vi "6b8pointdft.vi"() -> ()   [LabVIEW 2013]
uses:
  <vilib>/Analysis/2dsp.llb/Real FFT.vi
  <vilib>/Analysis/NI_AALPro.lvlib
panel:
  out "XY Graph":cluster{i32[], dbl[]}(graph)
  out "Waveform Graph 1+2":dynamicdata(graph)
  out "Waveform Graph 2":dynamicdata(graph)
  out "Waveform Graph 1":dynamicdata(graph)
  in  "Amplitude 2":dbl=1.0 caption="Amplitude"
  in  "Frequency 2":dbl=10.1 caption="Frequency"
  in  "Frequency":dbl=10.1
  in  "Amplitude":dbl=1.0
  # "G SURESH\n23A91A0417\nECE-A"
  # "6B) FAST FOURIER TRANSFROM"
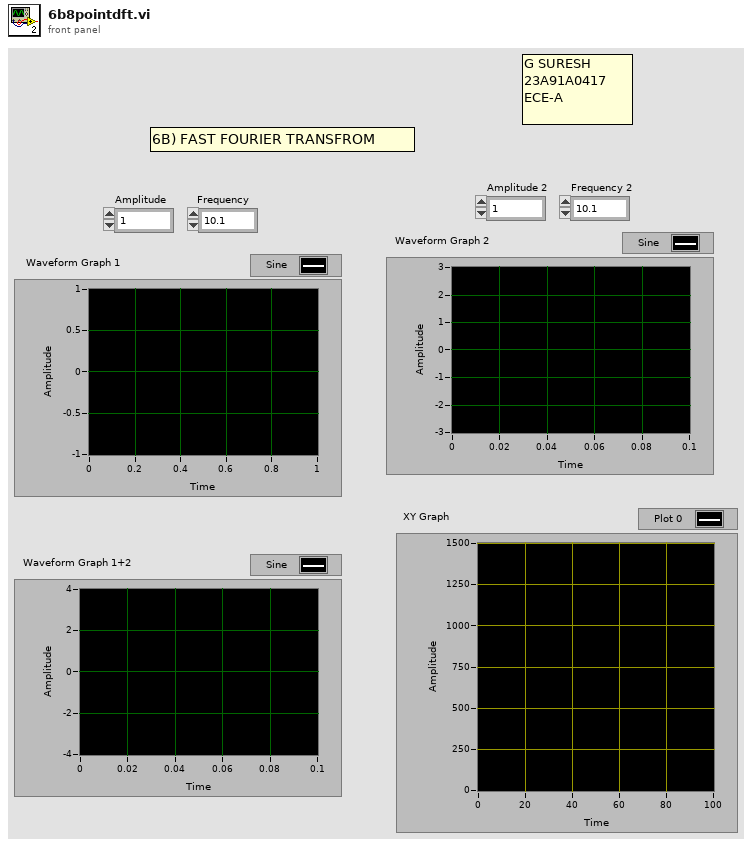
[diagram p1: front panel]
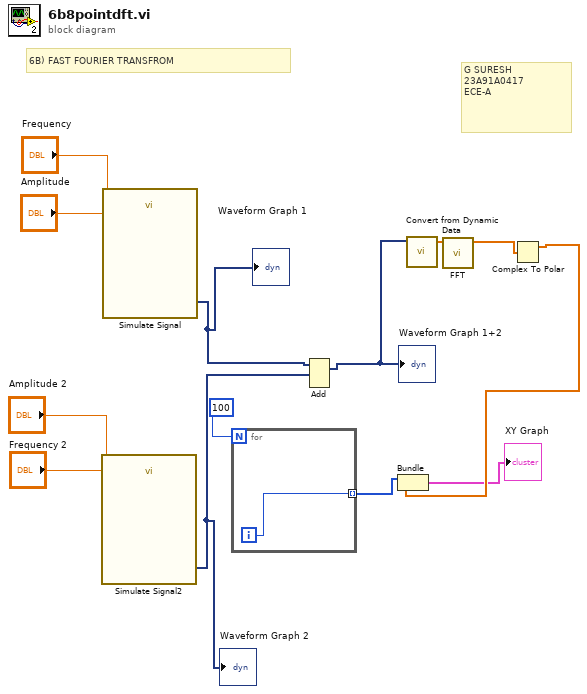
[diagram p0: block diagram]
diagram:
  # "6B) FAST FOURIER TRANSFROM"
  # "G SURESH\n23A91A0417\nECE-A"
  n1 = call "Simulate Signal2"("Frequency"="Frequency 2", "Amplitude"="Amplitude 2") -> ("Sine"=w9:dynamicdata)  [unwired: 12 in, 1 out]
  "Waveform Graph 2" <- w9
  n2 = call "Simulate Signal"("Frequency"="Frequency", "Amplitude"="Amplitude") -> ("Sine"=w8:dynamicdata)  [unwired: 12 in, 1 out]
  "Waveform Graph 1" <- w8
  n3 = for {
    N: 100 -> [_]
    tunnel: [w14] -> w4 mode=indexing
    i -> [w14]
  }
  n4 = Add(1:w9, 2:w8) -> (0:w7:dynamicdata)  [unwired: 1 in, 1 out]
  "Waveform Graph 1+2" <- w7
  n5 = call "Convert from Dynamic Data"("Dynamic Data Type"=w7) -> ("Array"=w6:dbl[])  [unwired: 3 in]
  n6 = call-poly <vilib>:"FFT.vi"("X"=w6) -> ("FFT {X}"=w3:cdb[])  [unwired: 9 in, 1 out]
  n7 = Complex To Polar(r * e^(i*theta)=w3) -> (r=w2:dbl[])  [unwired: 1 out]
  n8 = Bundle(w4, w2) -> (→"XY Graph":cluster{i32[], dbl[]})  [unwired: 1 in]
